vi "GetSelectedTag.vi"(10 "Tree in":refnum<class "Tree.lvclass">) -> (0 "error out":errorcluster, 2 "Selected Tag":string, 3 "Tree out":refnum<class "Tree.lvclass">)   [LabVIEW 2021, in "Tree.lvlib" / "Tree.lvclass"]
uses:
  Tree.lvclass
  Tree.lvclass/Tree.ctl
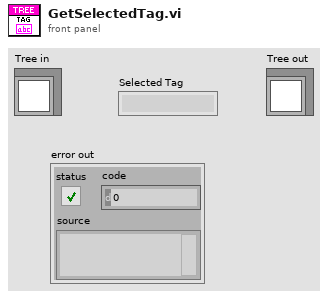
[diagram p1: front panel]
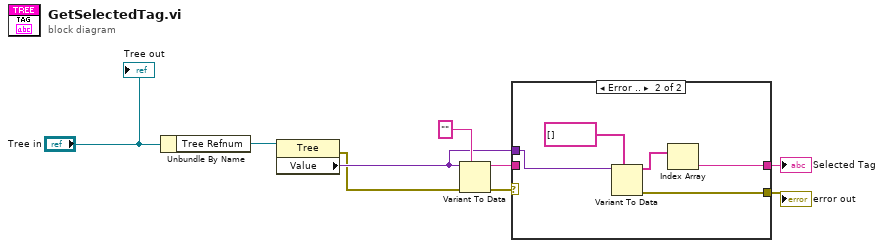
[diagram p0: block diagram]
diagram:
  n1 = Unbundle By Name("Tree in") -> ("Tree Refnum"=w8:refnum<vi>)
  n2 = property class="Tree"(reference=w8) -> (error out=w1:errorcluster, "Value"=w3:variant)  [unwired: 1 in, 1 out]
  n3 = Variant To Data(error in=w1, type="", Variant=w3) -> (data=w5:string, error out=w6:errorcluster)
  n4 = case shown="Error .." w6 {
    tunnel: w5 -> [w10 _]
    tunnel: [w10 w13] -> w4
    tunnel: w3 -> [_ w12]
    tunnel: [_ w11] -> w2
    frame No Error {
    }
    frame Error {
      n5 = Variant To Data(type=string[] [], Variant=w12) -> (data=w14:string[], error out=w11:errorcluster)  [unwired: 1 in]
      n6 = Index Array(array=w14) -> (element=w13:string)  [unwired: 1 in]
    }
  }
  "Selected Tag" <- w4
  "error out" <- w2
  "Tree out" <- "Tree in"
